vi "Test Instrument Framework.vi"   [LabVIEW 2019]
uses:
  lvsrc/SMOs/RemoteControl/Typedefs/RC Com Type--enum.ctl
  lvsrc/SMOs/RemoteControl/RemoteControl.lvclass
types:
  T1 = typedef "RemoteControl.lvclass/RC Com Type--enum.ctl" = enum16{"RC", "STM", "ZMQ"}
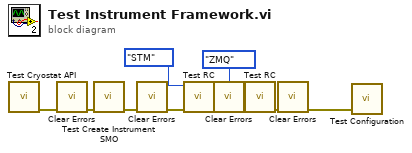
[diagram p0: block diagram]
diagram:
  n1 = call "Test Cryostat API.vi"() -> ("error out"=w5:errorcluster)  [unwired: 11 in]
  n2 = call <vilib>:"Clear Errors.vi"("error in (no error)"=w5) -> ("error out"=w4:errorcluster)  [unwired: 5 in, 1 out]
  n3 = call "Test Create Instrument SMO.vi"("error in (no error)"=w4) -> ("error out"=w6:errorcluster)  [unwired: 10 in]
  n4 = call <vilib>:"Clear Errors.vi"("error in (no error)"=w6) -> ("error out"=w2:errorcluster)  [unwired: 5 in, 1 out]
  n5 = call "Test RC.vi"("error in (no error)"=w2, "RC Type"=RC_Com_Type--enum."STM") -> ("error out"=w7:errorcluster)  [unwired: 9 in]
  n6 = call <vilib>:"Clear Errors.vi"("error in (no error)"=w7) -> ("error out"=w3:errorcluster)  [unwired: 5 in, 1 out]
  n7 = call "Test RC.vi"("error in (no error)"=w3, "RC Type"=RC_Com_Type--enum."ZMQ") -> ("error out"=w8:errorcluster)  [unwired: 9 in]
  n8 = call <vilib>:"Clear Errors.vi"("error in (no error)"=w8) -> ("error out"=w1:errorcluster)  [unwired: 5 in, 1 out]
  n9 = call "Test Configuration.vi"("error in (no error)"=w1) -> ()  [unwired: 10 in, 1 out]
